vi "Define Customized Character (5x10).vi"(8 "error in (no error)":errorcluster, 9 "customized character pattern":bool[][](array[boolean]), 10 "customized character code in":u8, 11 "LCD in":refnum<class "Character LCD.lvclass">) -> (0 "error out":errorcluster, 2 "customized character code out":u8, 3 "LCD out":refnum<class "Character LCD.lvclass">)   [LabVIEW 2015, in "HD44780 Host.lvlib"]
uses:
  HD44780 Host.lvlib
  Internal/LCD Class/Character LCD.lvclass
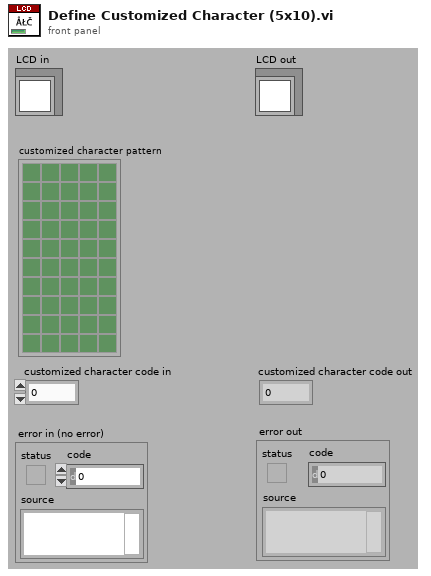
[diagram p1: front panel]
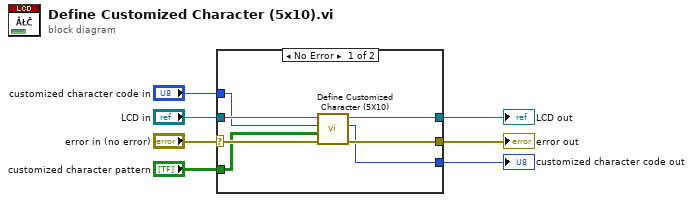
[diagram p0: block diagram]
diagram:
  n1 = case shown="No Error" "error in (no error)" {
    selector: "error in (no error)" -> [w14 w16]
    tunnel: [w12 w16] -> w6
    tunnel: "customized character pattern" -> [w9 _]
    tunnel: "customized character code in" -> [w10 _]
    tunnel: "LCD in" -> [w13 w15]
    tunnel: [w11 w15] -> w3
    tunnel: [w8 _] -> w1
    frame No Error {
      n2 = call-dynamic "Define Customized Character (5X10).vi"("error in (no error)"=w14, "customized character pattern"=w9, "customized character code in"=w10, "Character LCD in"=w13) -> ("error out"=w12:errorcluster, "customized character code out"=w8:u8, "Character LCD out"=w11:refnum<class "Character LCD.lvclass">)  [unwired: 5 in]
    }
    frame Error {
    }
  }
  "error out" <- w6
  "LCD out" <- w3
  "customized character code out" <- w1
